vi "Ejercicio_7_UART.vi"() -> ()   [LabVIEW 2021]
uses:
  <vilib>/Instr/_visa.llb/VISA Configure Serial Port (Instr).vi
panel:
  out "number":dbl
  out "min(x,y)":dbl
  out "max(x,y)":dbl
  in  "Rango \nmáximo":i32=75
  in  "Rango\nmínimo":i32=10
  out "Promedio":dbl
  out "Fuera de rango":bool
  in  "stop":bool
  in  "VISA resource name":refnum<visa-resource-name>
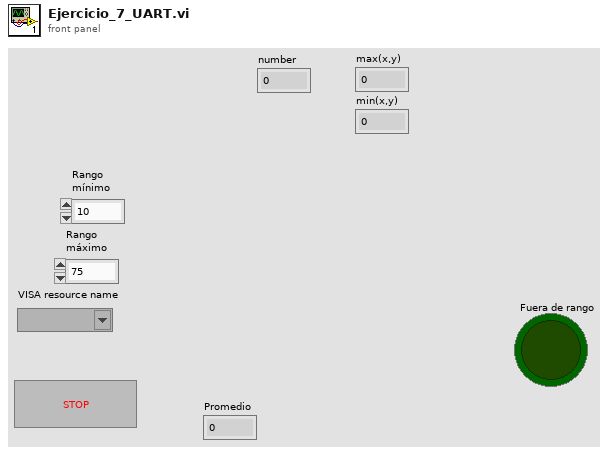
[diagram p1: front panel]
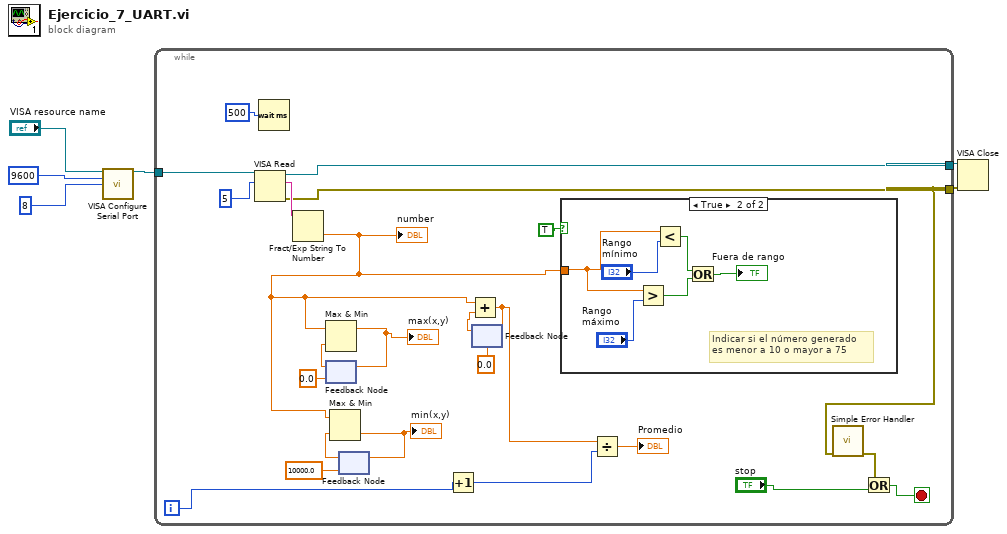
[diagram p0: block diagram]
diagram:
  n1 = call-poly "VISA Configure Serial Port"("VISA resource name"="VISA resource name", "baud rate (9600)"=u32 9600, "data bits (8)"=u16 8) -> ("VISA resource name out"=w3:refnum<visa-resource-name>)  [unwired: 11 in, 1 out]
  n2 = while {
    tunnel: w3 -> [w29]
    tunnel: [w26] -> w2
    tunnel: [w7] -> w1
    i -> [w21]
    stop <- w8 stop-if-true
    n3 = VISA Read(VISA resource name=w29, byte count=u32 5) -> (VISA resource name out=w26:refnum<visa-resource-name>, read buffer=w24:string, error out=w7:errorcluster)  [unwired: 1 in, 1 out]
    n4 = Wait (ms)(milliseconds to wait=u32 500) -> ()  [unwired: 1 out]
    n5 = Fract/Exp String To Number(string=w24) -> (number=w15:dbl)  [unwired: 3 in, 1 out]
    "number" <- w15
    n6 = feedback #1(0.0) -> (w17:dbl)
    n7 = Max & Min(x=w15, y=w17) -> (max(x,y)=w14:dbl)  [unwired: 1 out]
    "max(x,y)" <- w14
    n8 = feedback-in #1(w14) -> ()
    n9 = feedback #2(10000.0) -> (w13:dbl)
    n10 = Max & Min(x=w15, y=w13) -> (min(x,y)=w12:dbl)  [unwired: 1 out]
    "min(x,y)" <- w12
    n11 = feedback-in #2(w12) -> ()
    n12 = Increment(x=w21) -> (x+1=w23:i32)
    n13 = feedback #3(0.0) -> (w20:dbl)
    n14 = Add(x=w15, y=w20) -> (x+y=w19:dbl)
    n15 = feedback-in #3(w19) -> ()
    n16 = case shown="True" TRUE {
      tunnel: w15 -> [_ w35]
      frame False {
      }
      frame True {
        # "Indicar si el número generado \nes menor a 10 o mayor a 75"
        n17 = Greater?(x=w35, y="Rango \nmáximo") -> (0:w31:bool)
        n18 = Less?(x=w35, y="Rango\nmínimo") -> (x < y?=w32:bool)
        n19 = Or(x=w32, y=w31) -> (x .or. y?=→"Fuera de rango":bool)
      }
    }
    n20 = Divide(x=w19, y=w23) -> (x/y=→"Promedio":dbl)
    n21 = call <vilib>:"Simple Error Handler.vi"("error in (no error)"=w7) -> ("error out"=w10:errorcluster)  [unwired: 4 in, 4 out]
    n22 = Or(x=w10, y="stop") -> (x .or. y?=w8:bool)
  }
  n23 = VISA Close(VISA resource name=w2, error in (no error)=w1) -> ()  [unwired: 1 out]
